vi "Diagnostic Cycle.vi"(8 "error in (no error)":errorcluster, 11 "CAP-USB-1 in":refnum<class "CAP-USB-1.lvclass">) -> (0 "error out":errorcluster, 3 "CAP-USB-1 out":refnum<class "CAP-USB-1.lvclass">)   [LabVIEW 2014, in "CAP-USB-1.lvlib" / "CAP-USB-1.lvclass"]
doc: "Toma una Cantidad de muestras definidas Diagnostic Data.Muestras Diag. Cycle y las promedia"
uses:
  CAP-USB-1.lvclass
  CAP-USB-1.lvclass/CAP-USB-1.ctl
  API/CAP-USB/CAP-USB.lvlib
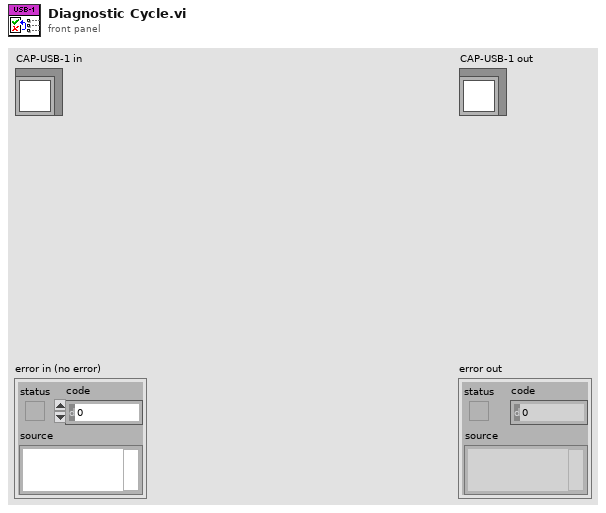
[diagram p1: front panel]
types:
  T1 = cluster{"Entradas":bool[], "Salidas":bool[], "Valor Encoder":u16, "Valor Transductores":u16[], "Orden Transd":u32[]}[]
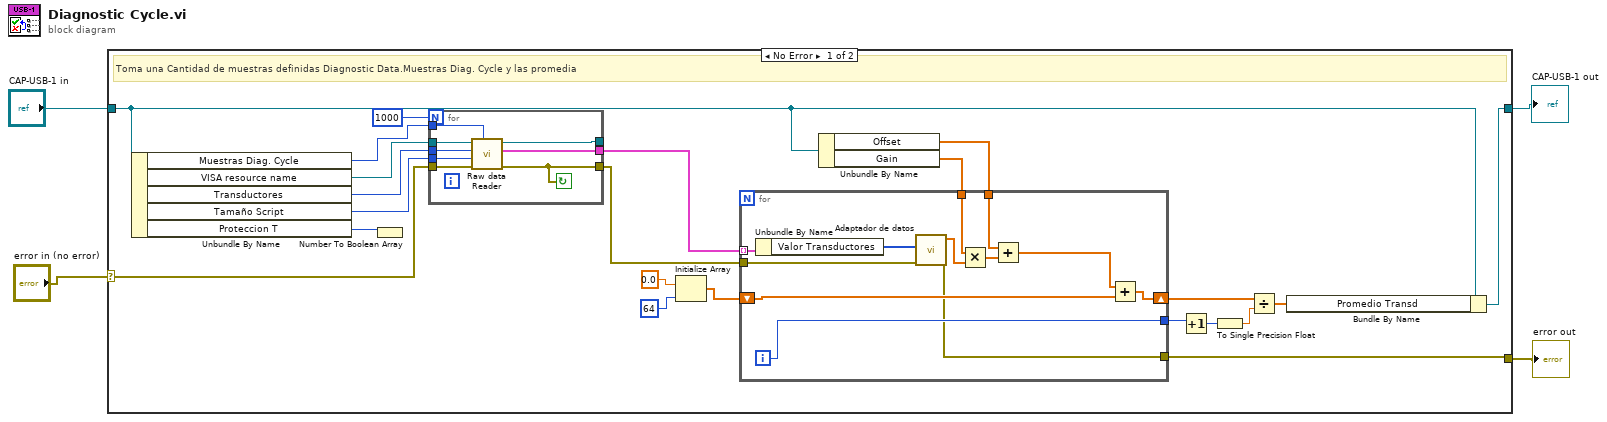
[diagram p0: block diagram]
diagram:
  n1 = case shown="No Error" "error in (no error)" {
    selector: "error in (no error)" -> [w16 w48]
    tunnel: [w17 w48] -> w3
    tunnel: [w11 w47] -> w1
    tunnel: "CAP-USB-1 in" -> [w7 w47]
    frame No Error {
      # "Toma una Cantidad de muestras definidas Diagnostic Data.Muestras Diag. Cycle y las promedia"
      n2 = Unbundle By Name(w7) -> ("Muestras Diag. Cycle"=w23:u32, "VISA resource name"=w26:refnum<visa-resource-name>, "Transductores"=w25:u64, "Tamaño Script"=w24:i32, "Proteccion T"=w9:u64)
      n3 = Number To Boolean Array(number=w9) -> ()  [unwired: 1 out]
      n4 = for {
        N: 1000 -> [_]
        tunnel: w26 -> [w34]
        tunnel: w25 -> [w33]
        tunnel: w24 -> [w32]
        tunnel: w23 -> [w31]
        tunnel: [w30] -> w13
        tunnel: w16 -> [w29]
        tunnel: [w28] -> w10
        tunnel: [w27] -> _
        stop <- w28 continue-if-true
        n5 = call "Raw data Reader.vi"("Num de tramas"=w31, "error in (no error)"=w29, "Tamaño Script"=w32, "TRANSDUCTORES"=w33, "VISA Refnum in"=w34) -> ("error out"=w28:errorcluster, "Raw data"=w30:T1, "VISA reference"=w27:refnum<visa-resource-name>)  [unwired: 2 in]
      }
      n6 = Initialize Array(sgl 0.0 ("Transductor"), 64 ("dimension size")) -> (w12:sgl[])
      n7 = Unbundle By Name(w7) -> ("Offset"=w5:sgl[], "Gain"=w6:sgl[])
      n8 = for {
        tunnel: w13 -> [w46] mode=indexing
        tunnel: w10 -> [w44]
        shift-right: [w42] -> w19
        shift-left: w12 -> [w43]
        tunnel: [w41] -> w22
        tunnel: [w40] -> w17
        tunnel: w6 -> [w39]
        tunnel: w5 -> [w37]
        i -> [w41]
        n9 = Unbundle By Name(w46) -> ("Valor Transductores"=w45:u16[])
        n10 = call "Adaptador de datos.vi"("error in (no error)"=w44, "Transductores"=w45) -> ("error out"=w40:errorcluster, "Transductores"=w36:sgl[])  [unwired: 7 in, 1 out]
        n11 = Multiply(x=w39, y=w36) -> (x*y=w38:sgl[])
        n12 = Add(x=w37, y=w38) -> (x+y=w35:sgl[])
        n13 = Add(x=w35, y=w43) -> (x+y=w42:sgl[])
      }
      n14 = Increment(x=w22) -> (x+1=w20:i32)
      n15 = To Single Precision Float(number=w20) -> (single precision float=w21:sgl)
      n16 = Divide(x=w19, y=w21) -> (x/y=w18:sgl[])
      n17 = Bundle By Name(cluster=w7, "Promedio Transd"=w18) -> (w11:refnum<class "CAP-USB-1.lvclass">)
    }
    frame Error {
    }
  }
  "error out" <- w3
  "CAP-USB-1 out" <- w1
